vi "Pcre2MatchDataOvector8.vi"(8 "error in":errorcluster, 9 "OvectorSize":u64, 10 "MatchDataSize":u64, 11 "pMatchData":u64 format="%.0x") -> (0 "error out":errorcluster, 2 "pOvector":u64 format="%.0x", 3 "pMatchData":u64 format="%.0x")   [LabVIEW 2021, in "libpcre2-8.lvlib"]
uses:
  libpcre2-8.lvlib
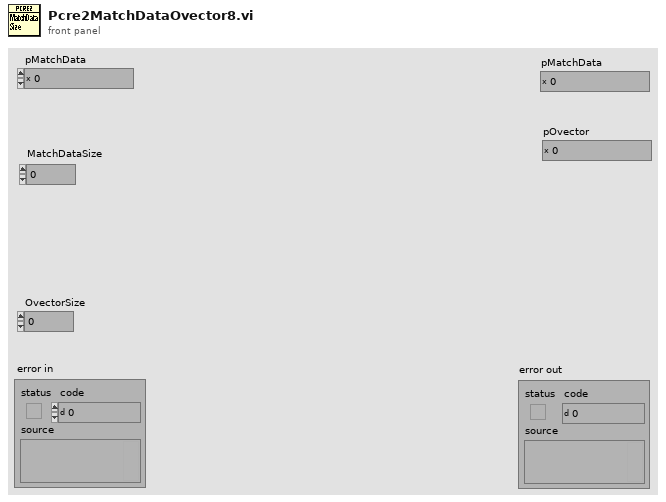
[diagram p1: front panel]
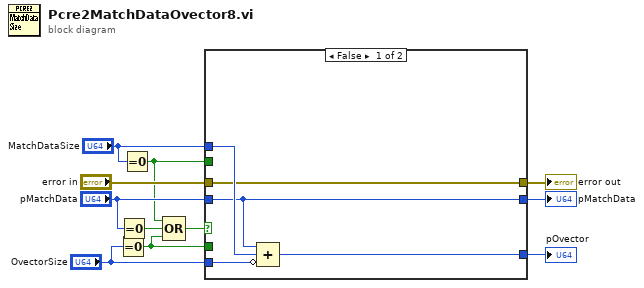
[diagram p0: block diagram]
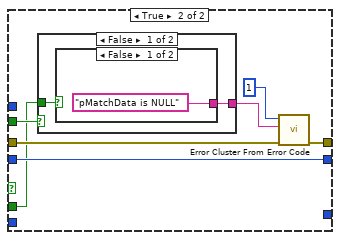
[diagram p2: hidden frame]
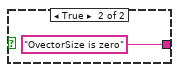
[diagram p3: hidden frame]
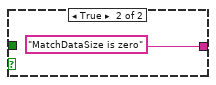
[diagram p4: hidden frame]
diagram:
  n1 = Equal To 0?(x="OvectorSize") -> (x = 0?=w3:bool)
  n2 = Equal To 0?(x="pMatchData") -> (x = 0?=w5:bool)
  n3 = Equal To 0?(x="MatchDataSize") -> (x = 0?=w1:bool)
  n4 = Compound Arithmetic op=OR(w1, w5, w3) -> (w4:bool)
  n5 = case shown="False" w4 {
    tunnel: "error in" -> [w13 w20]
    tunnel: [w13 w21] -> w10
    tunnel: "pMatchData" -> [w12 w23]
    tunnel: [w12 w23] -> w8
    tunnel: "OvectorSize" -> [w16 _]
    tunnel: [w15 _] -> w7
    tunnel: w3 -> [_ w18]
    tunnel: "MatchDataSize" -> [w14 _]
    tunnel: w1 -> [_ w19]
    frame False {
      n6 = Compound Arithmetic op=ADD(w12, w14, invert w16) -> (w15:u64)
    }
    frame True {
      n7 = case shown="False" w19 {
        tunnel: w18 -> [w25 _]
        tunnel: [w24 "MatchDataSize is zero" ("message")] -> w17
        frame False {
          n8 = case shown="False" w25 {
            tunnel: ["pMatchData is NULL" ("message") "OvectorSize is zero" ("message")] -> w24
            frame False {
            }
            frame True {
            }
          }
        }
        frame True {
        }
      }
      n9 = call <vilib>:"Error Cluster From Error Code.vi"("error in (no error)"=w20, "error message (\"\")"=w17, "error code (0)"=1 ("code (0)")) -> ("error out"=w21:errorcluster)  [unwired: 6 in]
    }
  }
  "pMatchData" <- w8
  "error out" <- w10
  "pOvector" <- w7
